vi "aft_Fixed-Point_Simulation_Template_(LMS).vi"(7 "reset":bool, 8 "error in (no error)":errorcluster, 9 "step size":fxp<+/-,16,-2>, 10 "d(n)":fxp<+/-,32,32>, 11 "x(n)":fxp<+/-,32,32>) -> (0 "error out":errorcluster, 1 "coefficient":fxp<+/-,16,1>[](array[numeric]), 2 "e(n)":fxp<+/-,24,1>, 3 "d'(n)":fxp<+/-,24,1>, 4 "simulation information":T1, 5 "fixed-point settings":T2={"algorithm"=0, "filter length"=128, "step size"=0.0999985, "encoding"={"x(n) word length"=24, "x(n) integer word length"=1, "d(n) word length"=24, "d(n) integer word length"=1, "w(n) word length"=24, "w(n) integer word length"=1, "step size word length"=16, "step size integer word length"=-2}} {"algorithm" items=["LMS"]})   [LabVIEW 2017]
uses:
  <vilib>/addons/Adaptive Filters/Utilities/AFT Fixed-Point Settings.ctl
  <vilib>/addons/Adaptive Filters/Utilities/AFT Simulation Info.ctl
  <vilib>/addons/Adaptive Filters/Utilities/AFT Algorithm.ctl
  <vilib>/addons/Adaptive Filters/NI_AdaptiveFilter.lvlib
panel:
  in  "dummy AFT fixed-point settings":T2={"algorithm"=0, "filter length"=128, "step size"=0.0999985, "encoding"={"x(n) word length"=24, "x(n) integer word length"=1, "d(n) word length"=24, "d(n) integer word length"=1, "w(n) word length"=24, "w(n) integer word length"=1, "step size word length"=16, "step size integer word length"=-2}} {"algorithm" items=["LMS"]}
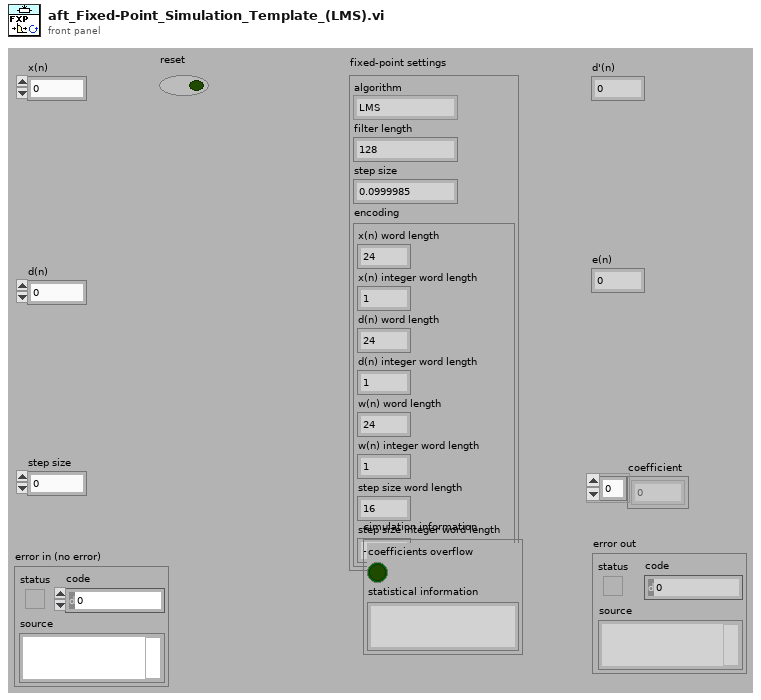
[diagram p1: front panel]
types:
  T1 = typedef "NI_AdaptiveFilter.lvlib/AFT Simulation Info.ctl" = cluster{"coefficients overflow":bool, "statistical information":string}
  T2 = typedef "NI_AdaptiveFilter.lvlib/AFT Fixed-Point Settings.ctl" = cluster{"algorithm":u16, "filter length":i32, "step size":dbl, "encoding":cluster{"x(n) word length":i32, "x(n) integer word length":i32, "d(n) word length":i32, "d(n) integer word length":i32, "w(n) word length":i32, "w(n) integer word length":i32, "step size word length":i32, "step size integer word length":i32}}
  T3 = cluster{"x(n) word length":i32, "x(n) integer word length":i32, "d(n) word length":i32, "d(n) integer word length":i32, "w(n) word length":i32, "w(n) integer word length":i32, "step size word length":i32, "step size integer word length":i32}
  T4 = typedef "NI_AdaptiveFilter.lvlib/AFT Algorithm.ctl" = u16
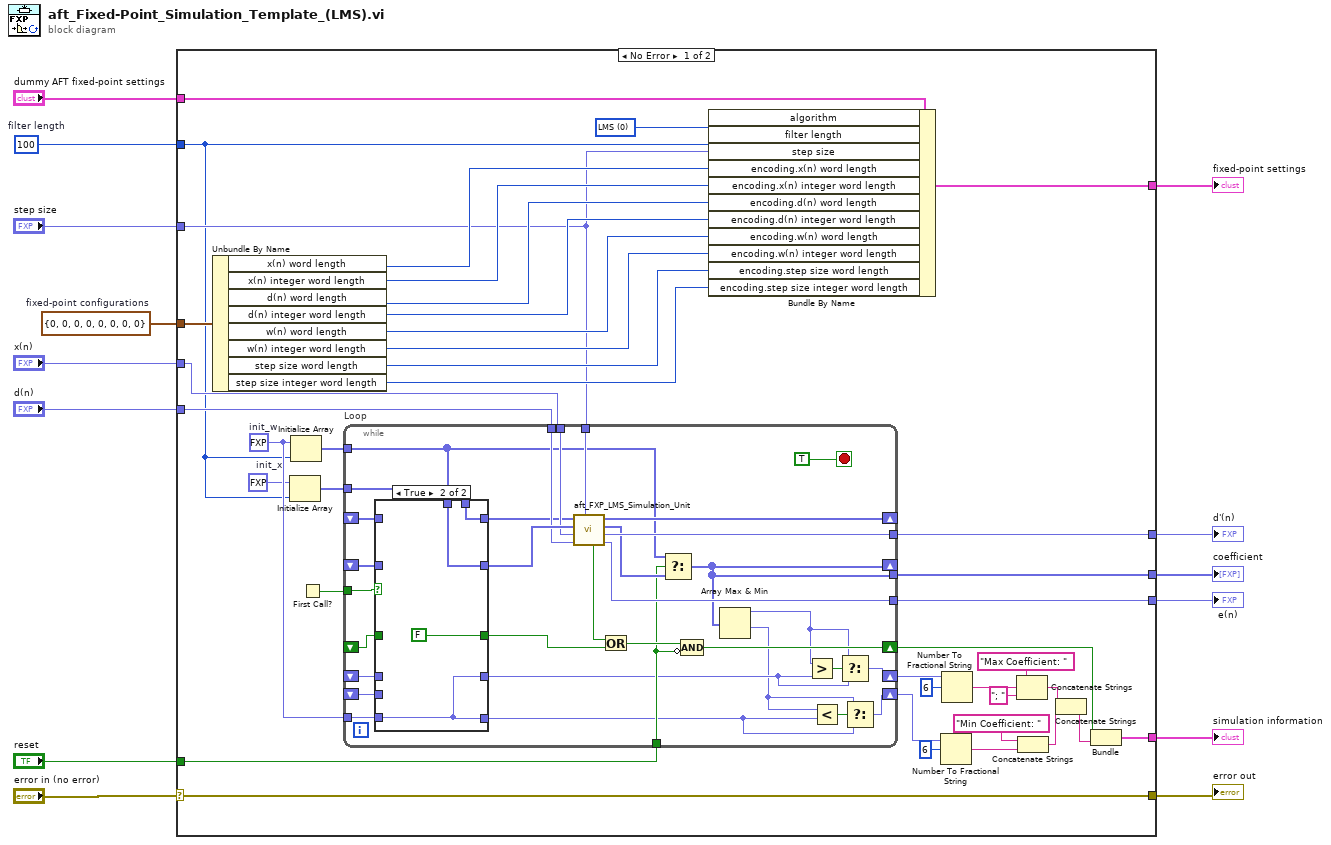
[diagram p0: block diagram]
diagram:
  w6 = T3 {"x(n) word length"=0, "x(n) integer word length"=0, "d(n) word length"=0, "d(n) integer word length"=0, "w(n) word length"=0, "w(n) integer word length"=0, "step size word length"=0, "step size integer word length"=0}  # fixed-point configurations
  w8 = 100  # filter length
  n1 = case "error" shown="No Error" "error in (no error)" {
    selector: "error in (no error)" -> [w52 w97]
    tunnel: "x(n)" -> [w23 _]
    tunnel: "d(n)" -> [w24 _]
    tunnel: [w22 _] -> w12
    tunnel: [w21 _] -> w11
    tunnel: [w39 _] -> w10
    tunnel: [w50 _] -> w2
    tunnel: "step size" -> [w18 _]
    tunnel: w8 -> [w16 _]
    tunnel: "reset" -> [w53 _]
    tunnel: w6 -> [w49 _]
    tunnel: [w52 w97] -> w4
    tunnel: "dummy AFT fixed-point settings" -> [w51 _]
    tunnel: [w37 _] -> w1
    frame No Error {
      w17 = fxp<+,1,1> 0.0  # init_x
      w19 = fxp<+,1,1> 0.0  # init_w
      w40 = T4 0 items=["LMS"] ("algorithm")
      n2 = Unbundle By Name(w49) -> ("x(n) word length"=w48:i32, "x(n) integer word length"=w47:i32, "d(n) word length"=w46:i32, "d(n) integer word length"=w45:i32, "w(n) word length"=w44:i32, "w(n) integer word length"=w43:i32, "step size word length"=w42:i32, "step size integer word length"=w41:i32)
      n3 = Initialize Array(w17, w16) -> (w15:fxp<+,1,1>[])
      n4 = Initialize Array(w19, w16) -> (w20:fxp<+,1,1>[])
      n5 = First Call?() -> (First Call?: T/F=w54:bool)
      n6 = while "Loop" {
        tunnel: w54 -> [w86]
        shift-right: [w82] -> _
        shift-left: _ -> [w85]
        shift-right: [w59] -> _
        shift-left: _ -> [w84]
        shift-right: [w70] -> w38
        shift-left: _ -> [w80]
        tunnel: w24 -> [w79]
        tunnel: [w75] -> w22
        tunnel: [w76] -> w21
        tunnel: w23 -> [w78]
        tunnel: w18 -> [w74]
        tunnel: w53 -> [w71]
        tunnel: [w59] -> w39
        shift-right: [w66] -> w36
        shift-left: _ -> [w61]
        shift-right: [w62] -> w30
        shift-left: _ -> [w60]
        tunnel: w20 -> [w58]
        tunnel: w19 -> [w57]
        tunnel: w15 -> [w55]
        stop <- TRUE stop-if-true
        n7 = case shown="True" w86 {
          tunnel: [w92 w93] -> w56
          tunnel: w85 -> [w92 _]
          tunnel: [w91 w94] -> w83
          tunnel: w84 -> [w91 _]
          tunnel: [w90 FALSE] -> w81
          tunnel: w80 -> [w90 _]
          tunnel: w58 -> [_ w94]
          tunnel: [w89 w95] -> w67
          tunnel: [w88 w95] -> w63
          tunnel: w61 -> [w89 _]
          tunnel: w60 -> [w88 _]
          tunnel: w57 -> [_ w95]
          tunnel: w55 -> [_ w93]
          frame False {
          }
          frame True {
          }
        }
        n8 = call <vilib>:"aft_FXP_LMS_Simulation_Unit.vi"("stepsize"=w74, "d(n)"=w79, "x(n)"=w78, "coefficients in"=w83, "state in"=w56) -> ("e(n)"=w76:fxp<+/-,32,32>, "d'(n)"=w75:fxp<+/-,32,16>, "coefficients out"=w73:fxp<+/-,64,81>[], "state out"=w82:fxp<+/-,32,32>[], "coefficients overflow"=w77:bool)  [unwired: 2 out]
        n9 = Or(x=w77, y=w81) -> (x .or. y?=w72:bool)
        n10 = Select(t=w58, s=w71, f=w73) -> (s? t:f=w59:fxp<+/-,64,81>[])
        n11 = Compound Arithmetic op=AND(w72, invert w71) -> (w70:bool)
        n12 = Array Max & Min(array=w59) -> (max value=w68:fxp<+/-,64,81>, min value=w64:fxp<+/-,64,81>)  [unwired: 2 out]
        n13 = Greater?(x=w68, y=w67) -> (0:w69:bool)
        n14 = Less?(x=w64, y=w63) -> (x < y?=w65:bool)
        n15 = Select(t=w68, s=w69, f=w67) -> (s? t:f=w66:fxp<+/-,64,81>)
        n16 = Select(t=w64, s=w65, f=w63) -> (s? t:f=w62:fxp<+/-,64,81>)
      }
      n17 = Bundle By Name(cluster=w51, "algorithm"=w40, "filter length"=w16, "step size"=w18, "encoding.x(n) word length"=w48, "encoding.x(n) integer word length"=w47, "encoding.d(n) word length"=w46, "encoding.d(n) integer word length"=w45, "encoding.w(n) word length"=w44, "encoding.w(n) integer word length"=w43, "encoding.step size word length"=w42, "encoding.step size integer word length"=w41) -> (w50:T2)
      n18 = Number To Fractional String(number=w30, width (-)=i16 6) -> (F-format string=w29:string)  [unwired: 2 out]
      n19 = Number To Fractional String(number=w36, width (-)=i16 6) -> (F-format string=w33:string)  [unwired: 2 out]
      n20 = Concatenate Strings("Max Coefficient: ", w33, "; " ("string")) -> (w25:string)
      n21 = Concatenate Strings("Min Coefficient: ", w29) -> (w28:string)
      n22 = Concatenate Strings(w25, w28) -> (w27:string)
      n23 = Bundle(w38, w27) -> (w37:cluster{bool, string})  [unwired: 1 out]
    }
    frame Error {
    }
  }
  "d'(n)" <- w12
  "e(n)" <- w11
  "coefficient" <- w10
  "error out" <- w4
  "fixed-point settings" <- w2
  "simulation information" <- w1
